vi "create_full_endpoint.vi"(8 "error in (no error)":errorcluster, 11 "llm_ollama_embedding in":refnum<class "llm_ollama_embedding.lvclass">) -> (0 "error out":errorcluster, 2 "endpoint":string, 3 "llm_ollama_embedding out":refnum<class "llm_ollama_embedding.lvclass">)   [LabVIEW 2020, in "llm_ollama_embedding.lvclass"]
uses:
  llm_ollama_embedding.lvclass
  llm_ollama_embedding.lvclass/llm_ollama_embedding.ctl
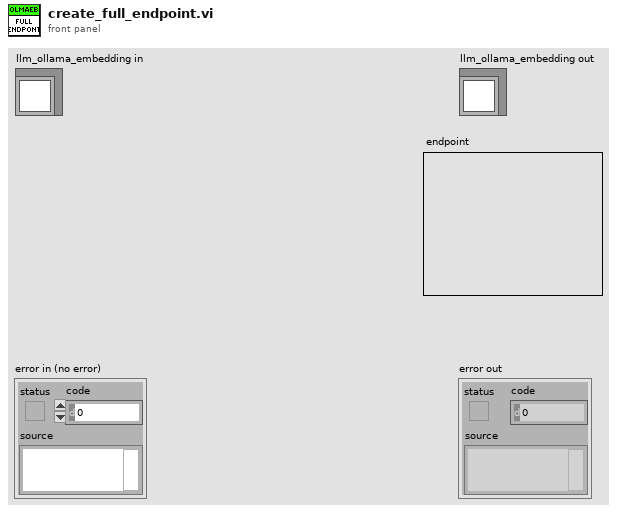
[diagram p1: front panel]
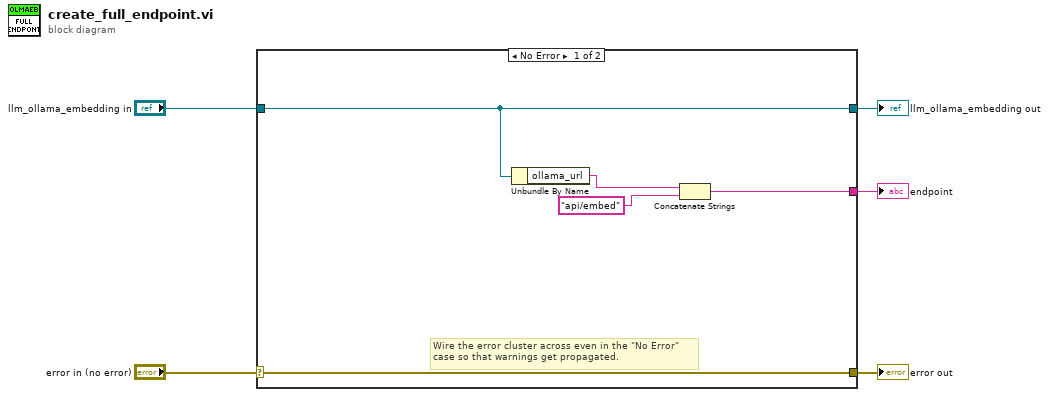
[diagram p0: block diagram]
diagram:
  n1 = case shown="No Error" "error in (no error)" {
    selector: "error in (no error)" -> [w10 w12]
    tunnel: [w10 w12] -> w4
    tunnel: [w8 w11] -> w2
    tunnel: "llm_ollama_embedding in" -> [w8 w11]
    tunnel: [w6 _] -> w1
    frame No Error {
      # "Wire the error cluster across even in the \"No Error\"\ncase so that warnings get propagated."
      n2 = Unbundle By Name(w8) -> ("ollama_url"=w7:string)
      n3 = Concatenate Strings(w7, "api/embed" ("url")) -> (w6:string)
    }
    frame Error {
    }
  }
  "error out" <- w4
  "llm_ollama_embedding out" <- w2
  "endpoint" <- w1
